vi "AM_Freq_Resp.vi"() -> ()   [LabVIEW 2019]
doc: "Use Arduino Micro and SparkFun MiniGen to measure Frequency Response of a Load\n\nR. Sheehan 18 - 11 - 2020"
uses:
  Build_Array.vi
  <vilib>/Instr/_visa.llb/VISA Configure Serial Port (Instr).vi
  <vilib>/measure/matone.llb/Extract Multiple Tone Information 1 Chan.vi
  <vilib>/measure/NI_MAPro.lvlib
panel:
  in  "Tab Control":T1(tab)
  in  "Addr":refnum<visa-resource-name>
  in  "Open Comms":bool
  out "Addr 2":refnum<visa-resource-name>
  out "Open":bool
  in  "Write f":bool
  in  "Frequency / Hz":dbl min=0.0 max=3.3
  in  "Delay (ms)":u32
  out "Cmd":string
  in  "Nreads":i32
  in  "Read":bool
  out "Meas / V":dbl[](array[numeric])
  out "Err / V":dbl[](array[numeric])
  out "Buffer Size":i32
  out "Buffer Data 2":string[](array[string])
  in  "fdelta / kHz":dbl
  in  "fhigh / kHz":dbl
  in  "flow / kHz":dbl
  in  "Sweep Meas.":bool
  out "XY Graph":cluster{dbl[], dbl[]}(graph)
  out "SmplData":cluster{"Times":dbl[], "Numerical Array":dbl[]}(graph)
  out "Tsmpl / us":i32
  in  "Sample":bool
  out "Nsmpl":i32
  out "Tones":T2(array[cluster]) {"detected phase (deg)" format="%_6g"; "detected amplitude" format="%_6p"; "detected frequency" format="%_6p"}
  out "Tsmpl / ms":dbl
  out "error out":errorcluster
  in  "Stop":bool
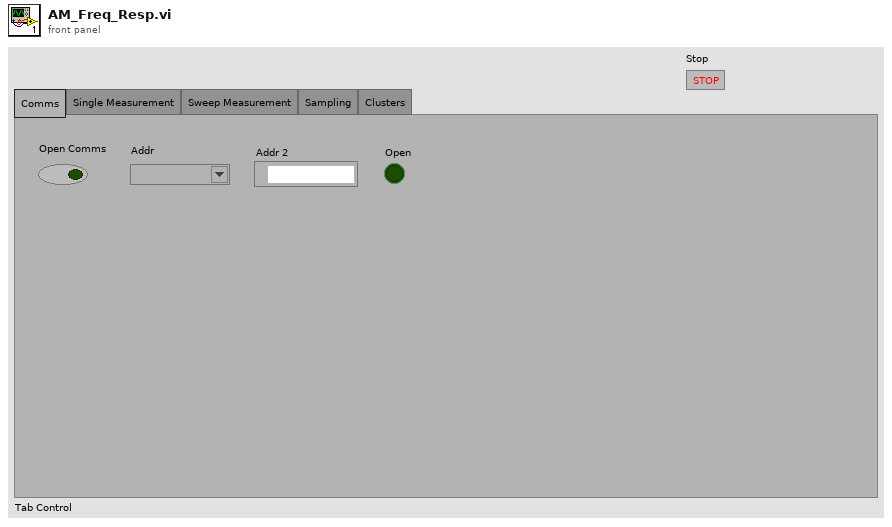
[diagram p1: front panel]
types:
  T1 = enum32{"Comms", "Single Measurement", "Sweep Measurement", "Sampling", "Clusters"}
  T2 = cluster{"detected frequency":dbl, "detected amplitude":dbl, "detected phase (deg)":dbl}[]
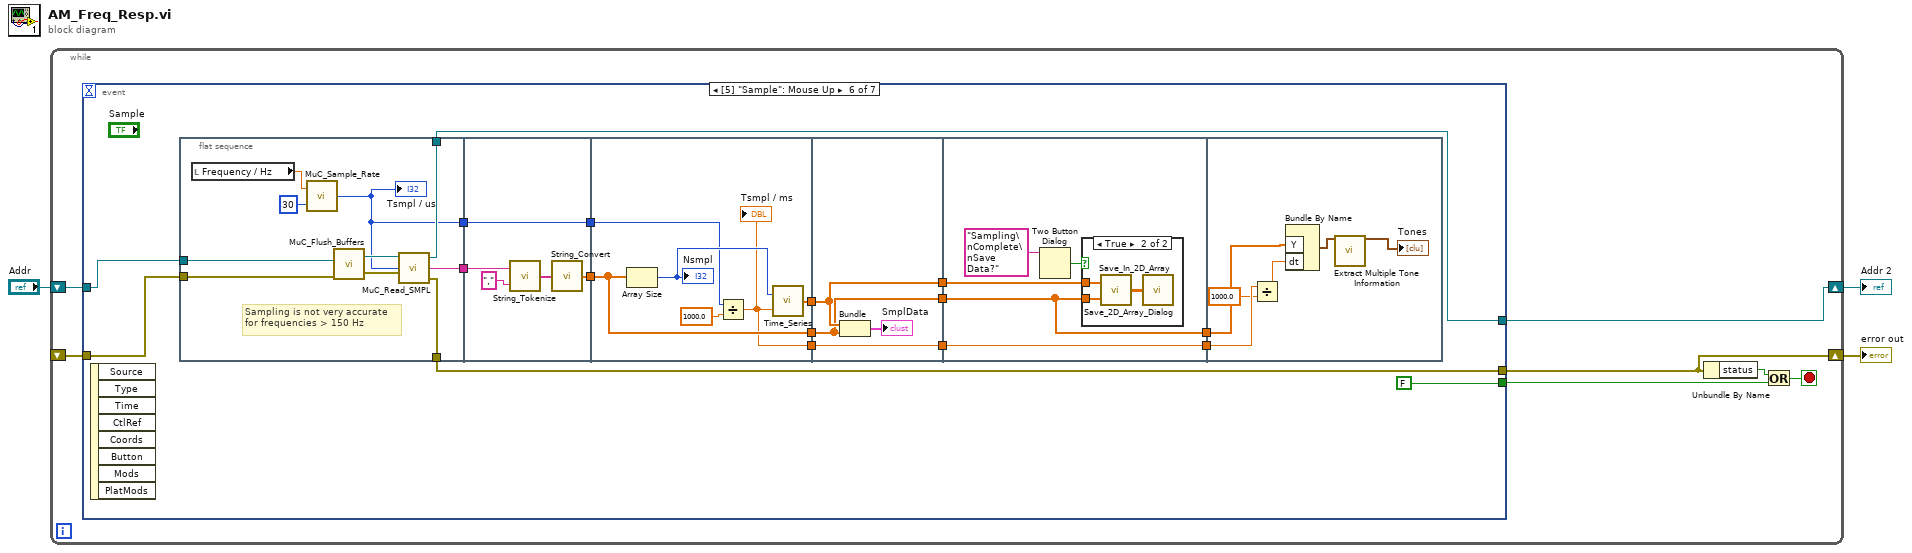
[diagram p0: block diagram]
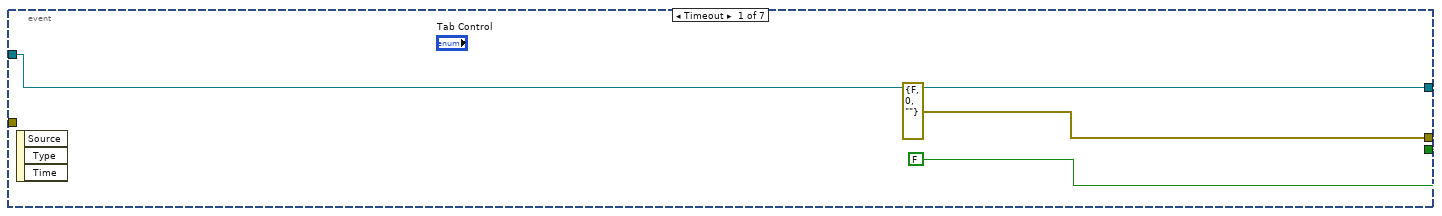
[diagram p2: hidden frame]
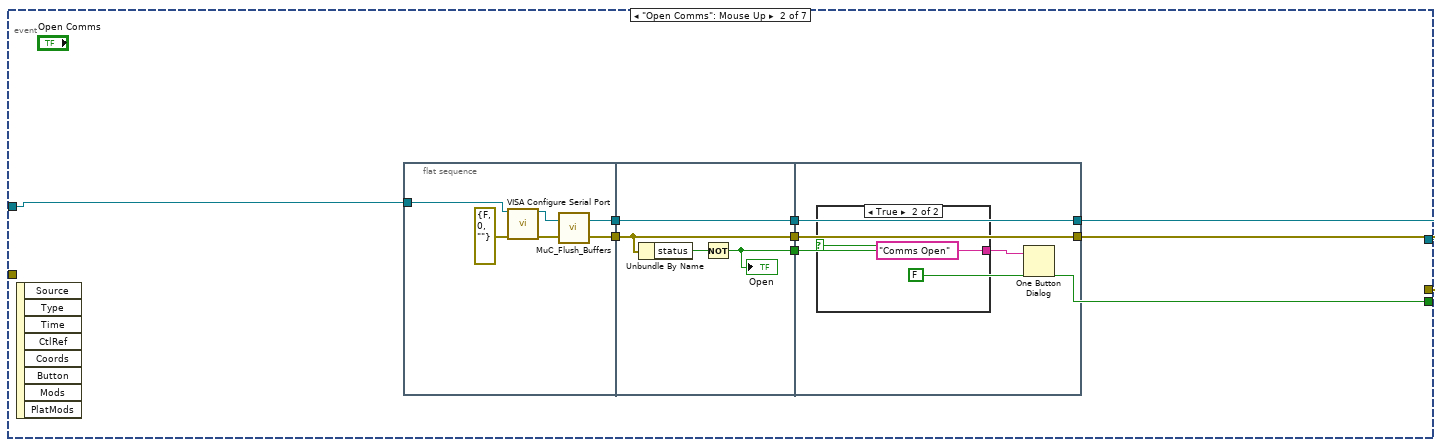
[diagram p3: hidden frame]
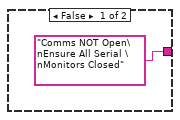
[diagram p4: hidden frame]
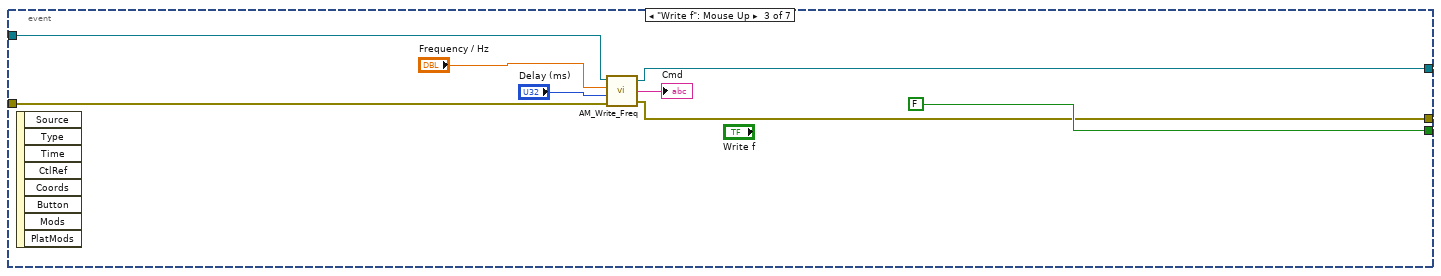
[diagram p5: hidden frame]
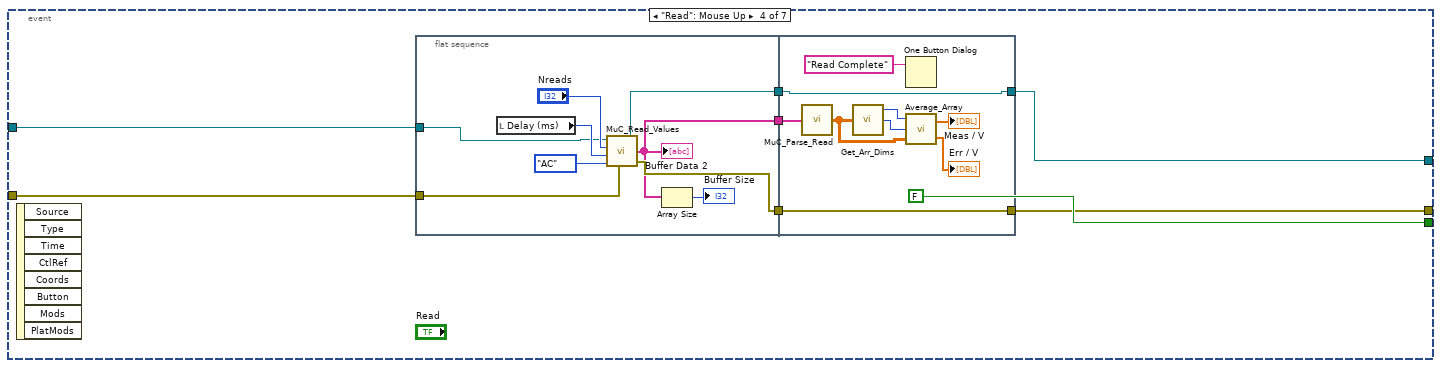
[diagram p6: hidden frame]
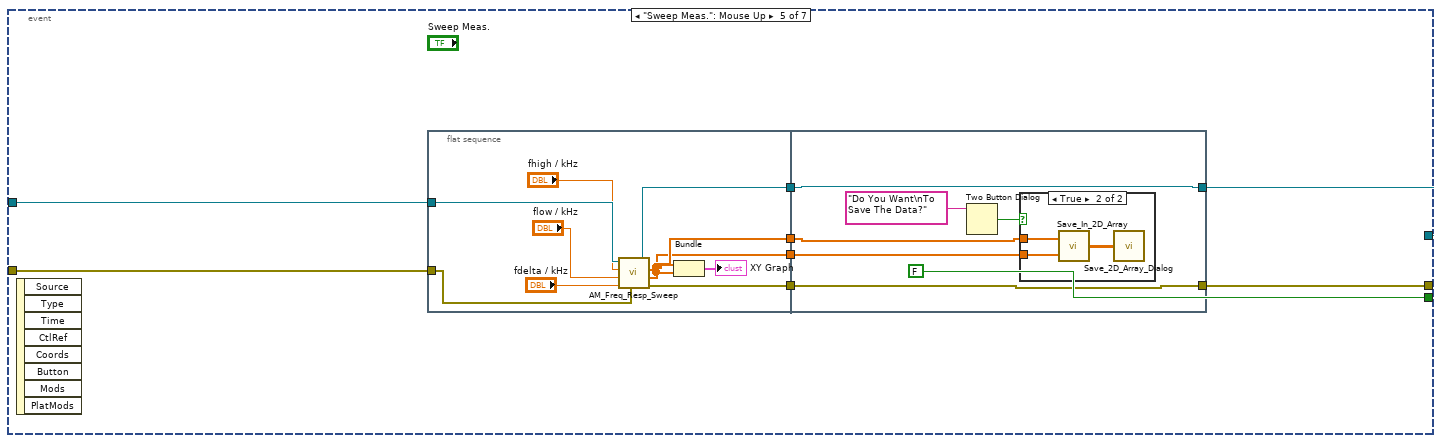
[diagram p7: hidden frame]
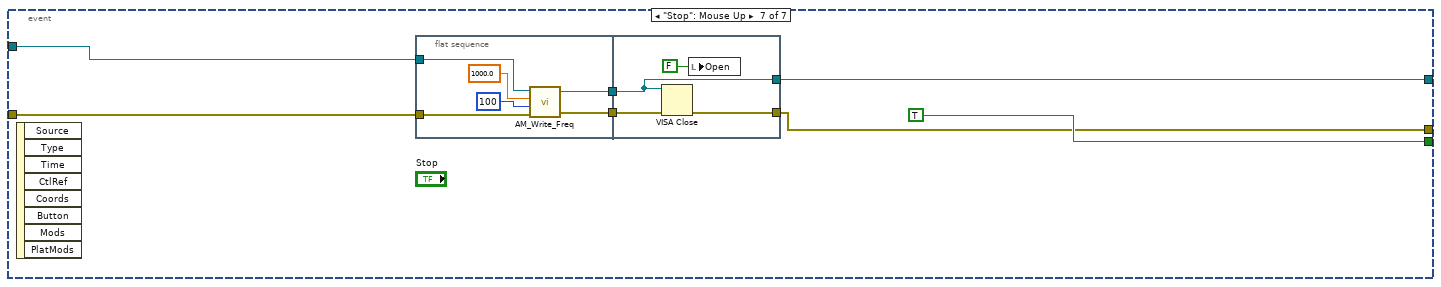
[diagram p10: hidden frame]
diagram:
  n1 = while {
    shift-right: [w9] -> w2
    shift-left: "Addr" -> [w10]
    shift-right: [w8] -> w1
    shift-left: _ -> [w7]
    stop <- w5 stop-if-true
    n2 = event shown="[5] \"Sample\": Mouse Up" {
      selector: _ -> [_ _ _ _ _ _ _]
      dyn-events: _ -> [_ _ _ _ _ _ _]
      timeout: _ -> [_ _ _ _ _ _ _]
      tunnel: w10 -> [w11 w22 w45 w53 w79 w110 w160]
      tunnel: [w11 w20 w42 w51 w78 w108 w158] -> w9
      tunnel: [errorcluster {"status"=FALSE, "code"=0, "source"=""} ("error in (no error)") w17 w41 w50 w77 w107 w162] -> w8
      tunnel: w7 -> [_ _ w44 w52 w80 w109 w161]
      tunnel: [FALSE FALSE FALSE FALSE FALSE FALSE TRUE] -> w4
      event Timeout {
        n3 = event-data() -> ()  [unwired: 1 in, 3 out]
      }
      event "Open Comms": Mouse Up {
        n4 = event-data() -> ()  [unwired: 1 in, 8 out]
        n5 = flat-sequence {
          tunnel: w22 -> [w27]
          tunnel: [w25] -> w19
          tunnel: [w23] -> w18
          tunnel: w19 -> [w32]
          tunnel: w18 -> [w31]
          tunnel: [w32] -> w16
          tunnel: [w31] -> w15
          tunnel: [w29] -> w14
          tunnel: [w35] -> w17
          tunnel: [w36] -> w20
          tunnel: w16 -> [w36]
          tunnel: w15 -> [w35]
          tunnel: w14 -> [w34]
          frame #0 {
            n6 = call-poly "VISA Configure Serial Port"("VISA resource name"=w27, "error in (no error)"=errorcluster {"status"=FALSE, "code"=0, "source"=""}) -> ("VISA resource name out"=w26:refnum<visa-resource-name>, "error out"=w24:errorcluster)  [unwired: 7 in, 5 out]
            n7 = call "MuC_Flush_Buffers.vi"("error in (no error)"=w24, "VISA resource name"=w26) -> ("error out"=w23:errorcluster, "VISA resource name 2"=w25:refnum<visa-resource-name>)
          }
          frame #1 {
            n8 = Unbundle By Name(w31) -> ("status"=w30:bool)
            n9 = Not(x=w30) -> (.not. x?=w29:bool)
            "Open" <- w29
          }
          frame #2 {
            n10 = case shown="True" w34 {
              tunnel: ["Comms NOT Open\nEnsure All Serial \nMonitors Closed" ("message") "Comms Open" ("message")] -> w33
              frame False {
              }
              frame True {
              }
            }
            n11 = One Button Dialog(message=w33) -> ()  [unwired: 1 in, 1 out]
          }
        }
      }
      event "Write f": Mouse Up {
        n12 = event-data() -> ()  [unwired: 1 in, 8 out]
        n13 = call "AM_Write_Freq.vi"("error in (no error)"=w44, "Delay / ms"="Delay (ms)", "f / Hz"="Frequency / Hz", "VISA resource name"=w45) -> ("error out"=w41:errorcluster, "Cmd"=→"Cmd":string, "VISA resource name 2"=w42:refnum<visa-resource-name>)
      }
      event "Read": Mouse Up {
        n14 = event-data() -> ()  [unwired: 1 in, 8 out]
        n15 = flat-sequence {
          tunnel: w53 -> [w58]
          tunnel: w52 -> [w57]
          tunnel: [w63] -> w49
          tunnel: [w62] -> w48
          tunnel: [w56] -> w47
          tunnel: [w71] -> w50
          tunnel: [w72] -> w51
          tunnel: w49 -> [w72]
          tunnel: w48 -> [w71]
          tunnel: w47 -> [w64]
          frame #0 {
            n16 = local read "Delay (ms)"() -> (w61:u32)
            n17 = call "MuC_Read_Values.vi"("VISA resource name"=w58, "Nreads"="Nreads", "Delay (ms)"=w61, "Read Type"=enum16{"DC", "AC"}."AC", "error in (no error)"=w57) -> ("VISA resource name 2"=w63:refnum<visa-resource-name>, "Buffer Data"=w56:string[], "error out"=w62:errorcluster)
            "Buffer Data 2" <- w56
            n18 = Array Size(array=w56) -> (size(s)=→"Buffer Size":i32)
          }
          frame #1 {
            n19 = call "MuC_Parse_Read.vi"("Buffer Data"=w64) -> ("Data"=w67:dbl[][])
            n20 = call "Get_Arr_Dims.vi"("Data"=w67) -> ("N Rows"=w66:i32, "N Cols"=w65:i32)  [unwired: 1 out]
            n21 = One Button Dialog(message="Read Complete") -> ()  [unwired: 1 in, 1 out]
            n22 = call "Average_Array.vi"("Array"=w67, "Ncolumns"=w65, "Nrows"=w66) -> ("Max-Min"=→"Err / V":dbl[], "Average"=→"Meas / V":dbl[])
          }
        }
      }
      event "Sweep Meas.": Mouse Up {
        n23 = event-data() -> ()  [unwired: 1 in, 8 out]
        n24 = flat-sequence {
          tunnel: w80 -> [w91]
          tunnel: w79 -> [w90]
          tunnel: [w89] -> w76
          tunnel: [w88] -> w75
          tunnel: [w83] -> w74
          tunnel: [w82] -> w73
          tunnel: [w96] -> w77
          tunnel: [w97] -> w78
          tunnel: w76 -> [w97]
          tunnel: w75 -> [w96]
          tunnel: w74 -> [w93]
          tunnel: w73 -> [w92]
          frame #0 {
            n25 = call "AM_Freq_Resp_Sweep.vi"("error in"=w91, "fdelta / kHz"="fdelta / kHz", "flow / kHz"="flow / kHz", "fhigh / kHz"="fhigh / kHz", "VISA resource name 2"=w90) -> ("error out"=w88:errorcluster, "Rdata"=w82:dbl[], "Fdata"=w83:dbl[], "VISA resource name 3"=w89:refnum<visa-resource-name>)
            n26 = Bundle("Fdata"=w83, "Rdata"=w82) -> (→"XY Graph":cluster{"Fdata":dbl[], "Rdata":dbl[]})  [unwired: 1 in]
          }
          frame #1 {
            n27 = Two Button Dialog(message="Do You Want\nTo Save The Data?") -> (T button?=w94:bool)  [unwired: 2 in]
            n28 = case shown="True" w94 {
              tunnel: w93 -> [_ w100]
              tunnel: w92 -> [_ w99]
              frame False {
              }
              frame True {
                n29 = call "Save_In_2D_Array.vi"("Vert"=w99, "Horz"=w100) -> ("Array"=w98:dbl[][])
                n30 = call "Save_2D_Array_Dialog.vi"("2D data"=w98) -> ()
              }
            }
          }
        }
      }
      event "Sample": Mouse Up {
        n31 = event-data() -> ()  [unwired: 1 in, 8 out]
        n32 = flat-sequence {
          tunnel: [w127] -> w116
          tunnel: w110 -> [w122]
          tunnel: w109 -> [w121]
          tunnel: [w126] -> w108
          tunnel: [w125] -> w107
          tunnel: [w118] -> w105
          tunnel: [w130] -> w115
          tunnel: w116 -> [w129]
          tunnel: [w128] -> w106
          tunnel: w105 -> [w128]
          tunnel: w115 -> [w135]
          tunnel: [w136] -> w114
          tunnel: [w135] -> w113
          tunnel: w106 -> [w134]
          tunnel: [w133] -> w101
          tunnel: w114 -> [w141]
          tunnel: w113 -> [w140]
          tunnel: [w141] -> w112
          tunnel: [w140] -> w111
          tunnel: [w139] -> w102
          tunnel: w101 -> [w139]
          tunnel: w112 -> [w145]
          tunnel: w111 -> [w144]
          tunnel: [w144] -> w104
          tunnel: [w143] -> w103
          tunnel: w102 -> [w143]
          tunnel: w104 -> [w156]
          tunnel: w103 -> [w155]
          frame #0 {
            # "Sampling is not very accurate\nfor frequencies > 150 Hz"
            n33 = local read "Frequency / Hz"() -> (w119:dbl)
            n34 = call "MuC_Sample_Rate.vi"("N smpls"=30, "Frequency / Hz"=w119) -> ("Sample Period / us"=w118:i32)
            "Tsmpl / us" <- w118
            n35 = call "MuC_Flush_Buffers.vi"("error in (no error)"=w121, "VISA resource name"=w122) -> ("error out"=w124:errorcluster, "VISA resource name 2"=w123:refnum<visa-resource-name>)
            n36 = call "MuC_Read_SMPL.vi"("error in (no error)"=w124, "Tsmpl / us"=w118, "VISA resource name"=w123) -> ("error out"=w125:errorcluster, "Cmd"=w127:string, "VISA resource name 2"=w126:refnum<visa-resource-name>)
          }
          frame #1 {
            n37 = call "String_Tokenize.vi"("String Token"=",", "String"=w129) -> ("String Array"=w132:string[])
            n38 = call "String_Convert.vi"("String Array"=w132) -> ("Numerical Array"=w130:dbl[])
          }
          frame #2 {
            n39 = Array Size(array=w135) -> (size(s)=w138:i32)
            "Nsmpl" <- w138
            n40 = Divide(x=w134, y=1000.0) -> (x/y=w133:dbl)
            "Tsmpl / ms" <- w133
            n41 = call "Time_Series.vi"("dt"=w133, "Nsmpls"=w138) -> ("Times"=w136:dbl[])
          }
          frame #3 {
            n42 = Bundle("Times"=w141, "Numerical Array"=w140) -> (→"SmplData":cluster{"Times":dbl[], "Numerical Array":dbl[]})  [unwired: 1 in]
          }
          frame #4 {
            n43 = Two Button Dialog(message="Sampling\nComplete\nSave Data?") -> (T button?=w147:bool)  [unwired: 2 in]
            n44 = case shown="True" w147 {
              tunnel: w145 -> [_ w149]
              tunnel: w144 -> [_ w148]
              frame False {
              }
              frame True {
                n45 = call "Save_In_2D_Array.vi"("Vert"=w148, "Horz"=w149) -> ("Array"=w150:dbl[][])
                n46 = call "Save_2D_Array_Dialog.vi"("2D data"=w150) -> ()
              }
            }
          }
          frame #5 {
            n47 = Divide(x=w155, y=1000.0) -> (x/y=w153:dbl)
            n48 = Bundle By Name("Y"=w156, "dt"=w153) -> (w152:waveform(dbl))  [unwired: 1 in]
            n49 = call-poly <vilib>:"Extract Multiple Tone Information.vi"("time signal in"=w152) -> ("multiple tone information"=→"Tones":T2)  [unwired: 12 in, 2 out]
          }
        }
      }
      event "Stop": Mouse Up {
        n50 = event-data() -> ()  [unwired: 1 in, 8 out]
        n51 = flat-sequence {
          tunnel: w161 -> [w166]
          tunnel: w160 -> [w169]
          tunnel: [w168] -> w159
          tunnel: [w167] -> w157
          tunnel: [w173] -> w162
          tunnel: w159 -> [w171]
          tunnel: [w171] -> w158
          tunnel: w157 -> [w170]
          frame #0 {
            n52 = call "AM_Write_Freq.vi"("error in (no error)"=w166, "Delay / ms"=u32 100, "f / Hz"=1000.0, "VISA resource name"=w169) -> ("error out"=w167:errorcluster, "VISA resource name 2"=w168:refnum<visa-resource-name>)  [unwired: 1 out]
          }
          frame #1 {
            n53 = VISA Close(VISA resource name=w171, error in (no error)=w170) -> (error out=w173:errorcluster)
            n54 = local write "Open"(FALSE) -> ()
          }
        }
      }
    }
    n55 = Unbundle By Name(w8) -> ("status"=w6:bool)
    n56 = Or(x=w6, y=w4) -> (x .or. y?=w5:bool)
  }
  "Addr 2" <- w2
  "error out" <- w1
